vi "Write Font.vi"(5 "Font":T1, 9 "Text in":refnum<class "Text.lvclass">) -> (3 "Text out":refnum<class "Text.lvclass">)   [LabVIEW 2014, in "Raspberry Pi Compatible Compiler for LabVIEW.lvlib" / "Text.lvclass"]
uses:
  Text.lvclass
  <vilib>/Utility/miscctls.llb/LVFontTypeDef.ctl
  Text.lvclass/Text.ctl
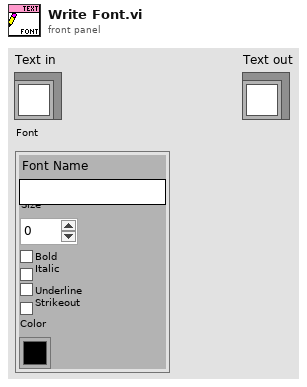
[diagram p1: front panel]
types:
  T1 = typedef "LVFontTypeDef.ctl" = cluster{"Font Name":string, "Size":u16, "Bold":bool, "Italic":bool, "Underline":bool, "Strikeout":bool, "Color":u32}
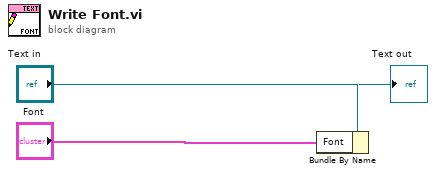
[diagram p0: block diagram]
diagram:
  n1 = Bundle By Name(cluster="Text in", "Font"="Font") -> (→"Text out":refnum<class "Text.lvclass">)
